vi "wondress graph.vi"() -> ()   [LabVIEW 2009]
panel:
  in  "stop":bool
  in  "index":i32(slide) scale=0.0..500.0
  out "Waveform Graph 2":waveform(i32)(graph)
  out "Progress 2":i32(slide) scale=-1.0..117.0
  out "Progress 1":i32(slide) scale=0.0..99.0
  out "Waveform Graph":i16[](graph)
  in  "range":i32
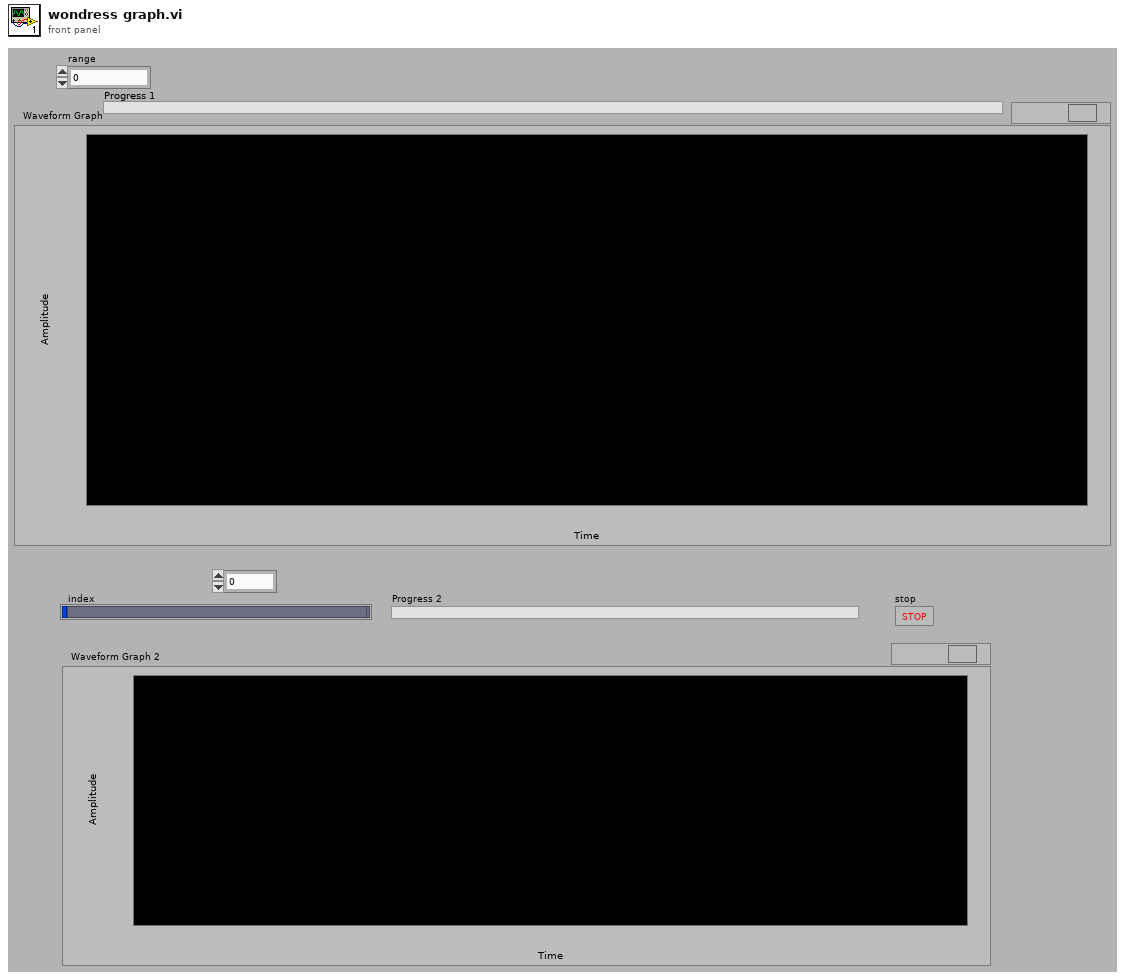
[diagram p1: front panel]
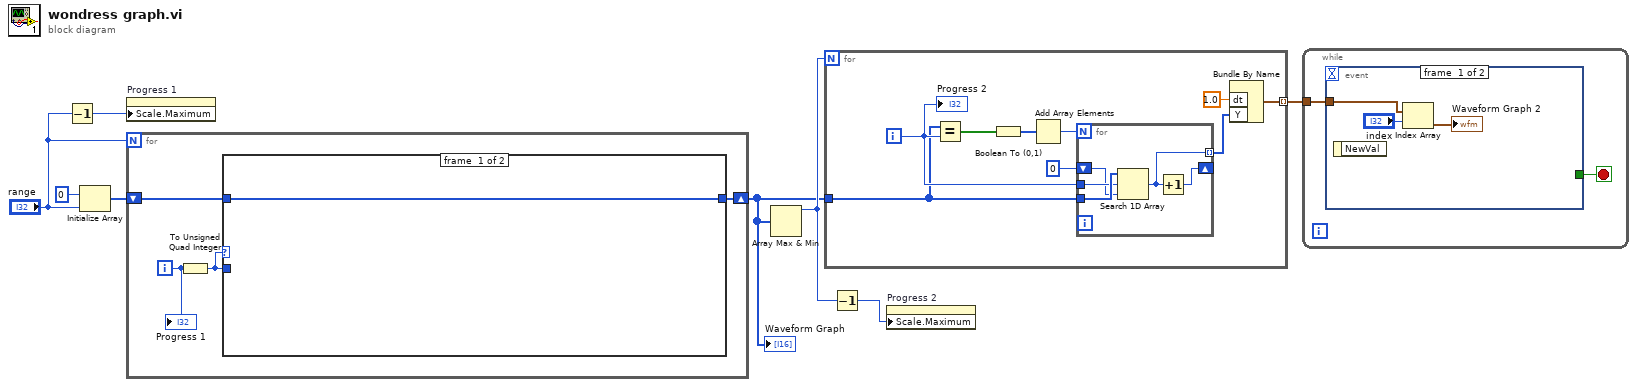
[diagram p0: block diagram]
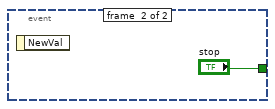
[diagram p2: hidden frame]
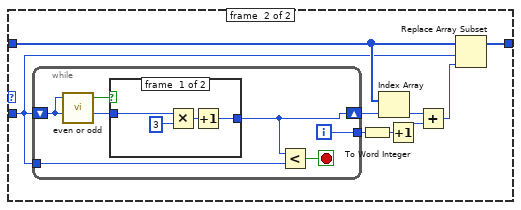
[diagram p3: hidden frame]
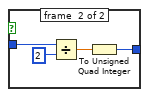
[diagram p4: hidden frame]
diagram:
  n1 = Decrement(x="range") -> (x-1=w2:i32)
  n2 = Initialize Array(i16 0 ("element"), "range") -> (w6:i16[])
  n3 = property on="Progress 1" class="Slide (strict)"("Scale.Maximum"=w2) -> ()  [unwired: 2 in, 2 out]
  n4 = for {
    N: "range" -> [_]
    shift-right: [w9] -> w4
    shift-left: w6 -> [w10]
    i -> [w12]
    n5 = To Unsigned Quad Integer(1:w12) -> (0:w11:u64)
    n6 = case shown="Default" w11 {
      tunnel: w11 -> [_ w16]
      tunnel: w10 -> [w13 w18]
      tunnel: [w13 w14] -> w9
      frame #0 {
      }
      frame #1 {
        n7 = while {
          tunnel: [w28] -> w22
          shift-right: [w25] -> w21
          shift-left: w16 -> [w26]
          tunnel: w16 -> [w23]
          i -> [w28]
          stop <- w24 stop-if-true
          n8 = call "even or odd.vi"("Numeric"=w26) -> ("Even?"=w27:bool)  [unwired: 4 in]
          n9 = case shown="False" w27 {
            tunnel: w26 -> [w29 w36]
            tunnel: [w31 w33] -> w25
            frame #0 {
              n10 = Multiply(x=w29, y=i64 3) -> (x*y=w30:u64)
              n11 = Increment(x=w30) -> (x+1=w31:u64)
            }
            frame #1 {
              n12 = Divide(x=w36, y=2) -> (x/y=w34:dbl)
              n13 = To Unsigned Quad Integer(1:w34) -> (0:w33:u64)
            }
          }
          n14 = Less?(x=w25, y=w23) -> (x < y?=w24:bool)
        }
        n15 = To Word Integer(number=w22) -> (16bit integer=w15:i16)
        n16 = Index Array(array=w18, index=w21) -> (element=w20:i16)
        n17 = Increment(x=w15) -> (x+1=w19:i16)
        n18 = Add(x=w20, y=w19) -> (x+y=w17:i16)
        n19 = Replace Array Subset(array=w18, new element=w17, index=w16) -> (w14:i16[])
      }
    }
    "Progress 1" <- w12
  }
  "Waveform Graph" <- w4
  n20 = Array Max & Min(array=w4) -> (max value=w5:i16)  [unwired: 3 out]
  n21 = for {
    N: w5 -> [_]
    tunnel: w4 -> [w43]
    tunnel: [w38] -> w1 mode=indexing
    i -> [w44]
    n22 = Equal?(x=w43, y=w44) -> (x = y?=w42:bool[])
    n23 = Boolean To (0,1)(Boolean=w42) -> (0, 1=w41:i16[])
    n24 = Add Array Elements(numeric array=w41) -> (sum=w40:i16)
    n25 = for {
      N: w40 -> [_]
      shift-right: [w46] -> _
      shift-left: 0 -> [w48]
      tunnel: w44 -> [w49]
      tunnel: w43 -> [w50]
      tunnel: [w47] -> w39 mode=indexing
      n26 = Search 1D Array(1D array=w50, element=w49, start index (0)=w48) -> (index of element=w47:i32)
      n27 = Increment(x=w47) -> (x+1=w46:i32)
    }
    n28 = Bundle By Name("dt"=1.0, "Y"=w39) -> (w38:waveform(i32))  [unwired: 1 in]
    "Progress 2" <- w44
  }
  n29 = Decrement(x=w5) -> (x-1=w3:i16)
  n30 = property on="Progress 2" class="Slide (strict)"("Scale.Maximum"=w3) -> ()  [unwired: 2 in, 2 out]
  n31 = while {
    tunnel: w1 -> [w52]
    stop <- w51 stop-if-true
    n32 = event shown="[1] \"stop\": Value Change" {
      selector: _ -> [_ _]
      dyn-events: _ -> [_ _]
      timeout: _ -> [_ _]
      tunnel: w52 -> [w55 _]
      tunnel: [_ "stop"] -> w51
      event #0 {
        n33 = event-data() -> ()  [unwired: 1 in, 1 out]
        n34 = Index Array(array=w55, index="index") -> (element=→"Waveform Graph 2":waveform(i32))
      }
      event #1 {
        n35 = event-data() -> ()  [unwired: 1 in, 1 out]
      }
    }
  }
